vi "6509 Sensor Inputs.vi"(2 "error in":errorcluster, 3 "Enum":T1(ring)) -> (0 "error out":errorcluster, 1 "State":bool)   [LabVIEW 2014]
panel:
  out "task out":refnum<k21>
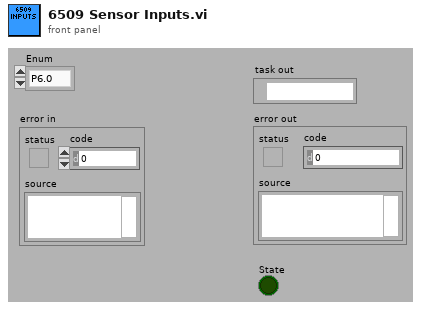
[diagram p1: front panel]
types:
  T1 = enum16{"P6.0", "P6.1", "P6.2", "P6.3", "P6.4", "P6.5", "P6.6", "P6.7", "P7.0", "P7.1", "P7.2", "P7.3", "P7.4", "P7.5", "P7.6", "P7.7", "P8.0", "P8.1", "P8.2", "P8.3", "P8.4", "P8.5", "P8.6", "P8.7", "P9.0", "P9.1", "P9.2", "P9.3", "P9.4", "P9.5", "P9.6", "P9.7", "11.0", "11.1", "11.2", "11.3", "11.4", "11.5", "11.6", "11.7", "Init"}
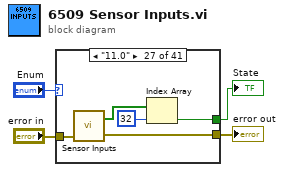
[diagram p0: block diagram]
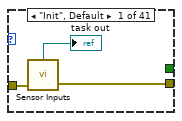
[diagram p2: hidden frame]
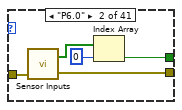
[diagram p3: hidden frame]
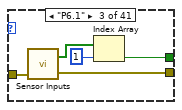
[diagram p4: hidden frame]
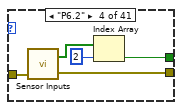
[diagram p5: hidden frame]
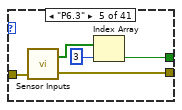
[diagram p6: hidden frame]
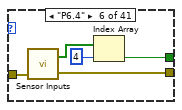
[diagram p7: hidden frame]
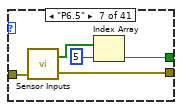
[diagram p8: hidden frame]
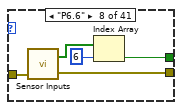
[diagram p9: hidden frame]
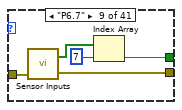
[diagram p10: hidden frame]
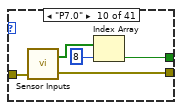
[diagram p11: hidden frame]
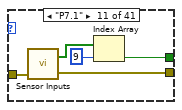
[diagram p12: hidden frame]
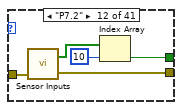
[diagram p13: hidden frame]
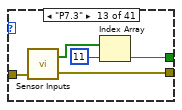
[diagram p14: hidden frame]
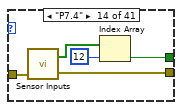
[diagram p15: hidden frame]
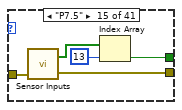
[diagram p16: hidden frame]
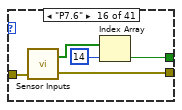
[diagram p17: hidden frame]
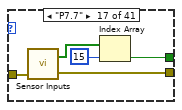
[diagram p18: hidden frame]
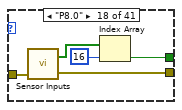
[diagram p19: hidden frame]
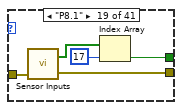
[diagram p20: hidden frame]
diagram:
  n1 = case shown="\"11.0\"" "Enum" {
    tunnel: "error in" -> [w7 w11 w15 w20 w23 w30 w35 w40 w45 w50 w55 w59 w65 w68 w75 w80 w85 w88 w95 w98 w103 w110 w113 w118 w123 w129 w134 w139 w144 w149 w154 w159 w164 w169 w175 w180 w184 w188 w194 w198 w204]
    tunnel: [w6 w10 w14 w19 w25 w28 w34 w39 w44 w49 w54 w60 w64 w70 w74 w79 w84 w90 w94 w100 w105 w109 w115 w120 w125 w130 w135 w140 w145 w150 w155 w160 w165 w170 w174 w179 w185 w190 w195 w200 w205] -> w2
    tunnel: [_ w8 w13 w18 w24 w29 w33 w38 w43 w48 w53 w58 w63 w69 w73 w78 w83 w89 w93 w99 w104 w108 w114 w119 w124 w128 w133 w138 w143 w148 w153 w158 w163 w168 w173 w178 w183 w189 w193 w199 w203] -> w1
    frame "Init", Default {
      n2 = call "Sensor Inputs.vi"("error in"=w7) -> ("error out"=w6:errorcluster, "task out"=→"task out":refnum<k21>)  [unwired: 2 in, 1 out]
    }
    frame "P6.0" {
      n3 = call "Sensor Inputs.vi"("error in"=w11) -> ("error out"=w10:errorcluster, "data"=w9:bool[])  [unwired: 2 in, 1 out]
      n4 = Index Array(array=w9, index=0) -> (element=w8:bool)
    }
    frame "P6.1" {
      n5 = call "Sensor Inputs.vi"("error in"=w15) -> ("error out"=w14:errorcluster, "data"=w16:bool[])  [unwired: 2 in, 1 out]
      n6 = Index Array(array=w16, index=1) -> (element=w13:bool)
    }
    frame "P6.2" {
      n7 = call "Sensor Inputs.vi"("error in"=w20) -> ("error out"=w19:errorcluster, "data"=w21:bool[])  [unwired: 2 in, 1 out]
      n8 = Index Array(array=w21, index=2) -> (element=w18:bool)
    }
    frame "P6.3" {
      n9 = call "Sensor Inputs.vi"("error in"=w23) -> ("error out"=w25:errorcluster, "data"=w26:bool[])  [unwired: 2 in, 1 out]
      n10 = Index Array(array=w26, index=3) -> (element=w24:bool)
    }
    frame "P6.4" {
      n11 = call "Sensor Inputs.vi"("error in"=w30) -> ("error out"=w28:errorcluster, "data"=w31:bool[])  [unwired: 2 in, 1 out]
      n12 = Index Array(array=w31, index=4) -> (element=w29:bool)
    }
    frame "P6.5" {
      n13 = call "Sensor Inputs.vi"("error in"=w35) -> ("error out"=w34:errorcluster, "data"=w36:bool[])  [unwired: 2 in, 1 out]
      n14 = Index Array(array=w36, index=5) -> (element=w33:bool)
    }
    frame "P6.6" {
      n15 = call "Sensor Inputs.vi"("error in"=w40) -> ("error out"=w39:errorcluster, "data"=w41:bool[])  [unwired: 2 in, 1 out]
      n16 = Index Array(array=w41, index=6) -> (element=w38:bool)
    }
    frame "P6.7" {
      n17 = call "Sensor Inputs.vi"("error in"=w45) -> ("error out"=w44:errorcluster, "data"=w46:bool[])  [unwired: 2 in, 1 out]
      n18 = Index Array(array=w46, index=7) -> (element=w43:bool)
    }
    frame "P7.0" {
      n19 = call "Sensor Inputs.vi"("error in"=w50) -> ("error out"=w49:errorcluster, "data"=w51:bool[])  [unwired: 2 in, 1 out]
      n20 = Index Array(array=w51, index=8) -> (element=w48:bool)
    }
    frame "P7.1" {
      n21 = call "Sensor Inputs.vi"("error in"=w55) -> ("error out"=w54:errorcluster, "data"=w56:bool[])  [unwired: 2 in, 1 out]
      n22 = Index Array(array=w56, index=9) -> (element=w53:bool)
    }
    frame "P7.2" {
      n23 = call "Sensor Inputs.vi"("error in"=w59) -> ("error out"=w60:errorcluster, "data"=w61:bool[])  [unwired: 2 in, 1 out]
      n24 = Index Array(array=w61, index=10) -> (element=w58:bool)
    }
    frame "P7.3" {
      n25 = call "Sensor Inputs.vi"("error in"=w65) -> ("error out"=w64:errorcluster, "data"=w66:bool[])  [unwired: 2 in, 1 out]
      n26 = Index Array(array=w66, index=11) -> (element=w63:bool)
    }
    frame "P7.4" {
      n27 = call "Sensor Inputs.vi"("error in"=w68) -> ("error out"=w70:errorcluster, "data"=w71:bool[])  [unwired: 2 in, 1 out]
      n28 = Index Array(array=w71, index=12) -> (element=w69:bool)
    }
    frame "P7.5" {
      n29 = call "Sensor Inputs.vi"("error in"=w75) -> ("error out"=w74:errorcluster, "data"=w76:bool[])  [unwired: 2 in, 1 out]
      n30 = Index Array(array=w76, index=13) -> (element=w73:bool)
    }
    frame "P7.6" {
      n31 = call "Sensor Inputs.vi"("error in"=w80) -> ("error out"=w79:errorcluster, "data"=w81:bool[])  [unwired: 2 in, 1 out]
      n32 = Index Array(array=w81, index=14) -> (element=w78:bool)
    }
    frame "P7.7" {
      n33 = call "Sensor Inputs.vi"("error in"=w85) -> ("error out"=w84:errorcluster, "data"=w86:bool[])  [unwired: 2 in, 1 out]
      n34 = Index Array(array=w86, index=15) -> (element=w83:bool)
    }
    frame "P8.0" {
      n35 = call "Sensor Inputs.vi"("error in"=w88) -> ("error out"=w90:errorcluster, "data"=w91:bool[])  [unwired: 2 in, 1 out]
      n36 = Index Array(array=w91, index=16) -> (element=w89:bool)
    }
    frame "P8.1" {
      n37 = call "Sensor Inputs.vi"("error in"=w95) -> ("error out"=w94:errorcluster, "data"=w96:bool[])  [unwired: 2 in, 1 out]
      n38 = Index Array(array=w96, index=17) -> (element=w93:bool)
    }
    frame "P8.2" {
      n39 = call "Sensor Inputs.vi"("error in"=w98) -> ("error out"=w100:errorcluster, "data"=w101:bool[])  [unwired: 2 in, 1 out]
      n40 = Index Array(array=w101, index=18) -> (element=w99:bool)
    }
    frame "P8.3" {
      n41 = call "Sensor Inputs.vi"("error in"=w103) -> ("error out"=w105:errorcluster, "data"=w106:bool[])  [unwired: 2 in, 1 out]
      n42 = Index Array(array=w106, index=19) -> (element=w104:bool)
    }
    frame "P8.4" {
      n43 = call "Sensor Inputs.vi"("error in"=w110) -> ("error out"=w109:errorcluster, "data"=w111:bool[])  [unwired: 2 in, 1 out]
      n44 = Index Array(array=w111, index=20) -> (element=w108:bool)
    }
    frame "P8.5" {
      n45 = call "Sensor Inputs.vi"("error in"=w113) -> ("error out"=w115:errorcluster, "data"=w116:bool[])  [unwired: 2 in, 1 out]
      n46 = Index Array(array=w116, index=21) -> (element=w114:bool)
    }
    frame "P8.6" {
      n47 = call "Sensor Inputs.vi"("error in"=w118) -> ("error out"=w120:errorcluster, "data"=w121:bool[])  [unwired: 2 in, 1 out]
      n48 = Index Array(array=w121, index=22) -> (element=w119:bool)
    }
    frame "P8.7" {
      n49 = call "Sensor Inputs.vi"("error in"=w123) -> ("error out"=w125:errorcluster, "data"=w126:bool[])  [unwired: 2 in, 1 out]
      n50 = Index Array(array=w126, index=23) -> (element=w124:bool)
    }
    frame "P9.0" {
      n51 = call "Sensor Inputs.vi"("error in"=w129) -> ("error out"=w130:errorcluster, "data"=w131:bool[])  [unwired: 2 in, 1 out]
      n52 = Index Array(array=w131, index=24) -> (element=w128:bool)
    }
    frame "11.0" {
      n53 = call "Sensor Inputs.vi"("error in"=w134) -> ("error out"=w135:errorcluster, "data"=w136:bool[])  [unwired: 2 in, 1 out]
      n54 = Index Array(array=w136, index=32) -> (element=w133:bool)
    }
    frame "11.1" {
      n55 = call "Sensor Inputs.vi"("error in"=w139) -> ("error out"=w140:errorcluster, "data"=w141:bool[])  [unwired: 2 in, 1 out]
      n56 = Index Array(array=w141, index=33) -> (element=w138:bool)
    }
    frame "11.2" {
      n57 = call "Sensor Inputs.vi"("error in"=w144) -> ("error out"=w145:errorcluster, "data"=w146:bool[])  [unwired: 2 in, 1 out]
      n58 = Index Array(array=w146, index=34) -> (element=w143:bool)
    }
    frame "11.3" {
      n59 = call "Sensor Inputs.vi"("error in"=w149) -> ("error out"=w150:errorcluster, "data"=w151:bool[])  [unwired: 2 in, 1 out]
      n60 = Index Array(array=w151, index=35) -> (element=w148:bool)
    }
    frame "11.4" {
      n61 = call "Sensor Inputs.vi"("error in"=w154) -> ("error out"=w155:errorcluster, "data"=w156:bool[])  [unwired: 2 in, 1 out]
      n62 = Index Array(array=w156, index=36) -> (element=w153:bool)
    }
    frame "11.5" {
      n63 = call "Sensor Inputs.vi"("error in"=w159) -> ("error out"=w160:errorcluster, "data"=w161:bool[])  [unwired: 2 in, 1 out]
      n64 = Index Array(array=w161, index=37) -> (element=w158:bool)
    }
    frame "11.6" {
      n65 = call "Sensor Inputs.vi"("error in"=w164) -> ("error out"=w165:errorcluster, "data"=w166:bool[])  [unwired: 2 in, 1 out]
      n66 = Index Array(array=w166, index=38) -> (element=w163:bool)
    }
    frame "11.7" {
      n67 = call "Sensor Inputs.vi"("error in"=w169) -> ("error out"=w170:errorcluster, "data"=w171:bool[])  [unwired: 2 in, 1 out]
      n68 = Index Array(array=w171, index=39) -> (element=w168:bool)
    }
    frame "P9.1" {
      n69 = call "Sensor Inputs.vi"("error in"=w175) -> ("error out"=w174:errorcluster, "data"=w176:bool[])  [unwired: 2 in, 1 out]
      n70 = Index Array(array=w176, index=25) -> (element=w173:bool)
    }
    frame "P9.2" {
      n71 = call "Sensor Inputs.vi"("error in"=w180) -> ("error out"=w179:errorcluster, "data"=w181:bool[])  [unwired: 2 in, 1 out]
      n72 = Index Array(array=w181, index=27) -> (element=w178:bool)
    }
    frame "P9.3" {
      n73 = call "Sensor Inputs.vi"("error in"=w184) -> ("error out"=w185:errorcluster, "data"=w186:bool[])  [unwired: 2 in, 1 out]
      n74 = Index Array(array=w186, index=28) -> (element=w183:bool)
    }
    frame "P9.4" {
      n75 = call "Sensor Inputs.vi"("error in"=w188) -> ("error out"=w190:errorcluster, "data"=w191:bool[])  [unwired: 2 in, 1 out]
      n76 = Index Array(array=w191, index=29) -> (element=w189:bool)
    }
    frame "P9.5" {
      n77 = call "Sensor Inputs.vi"("error in"=w194) -> ("error out"=w195:errorcluster, "data"=w196:bool[])  [unwired: 2 in, 1 out]
      n78 = Index Array(array=w196, index=30) -> (element=w193:bool)
    }
    frame "P9.6" {
      n79 = call "Sensor Inputs.vi"("error in"=w198) -> ("error out"=w200:errorcluster, "data"=w201:bool[])  [unwired: 2 in, 1 out]
      n80 = Index Array(array=w201, index=31) -> (element=w199:bool)
    }
    frame "P9.7" {
      n81 = call "Sensor Inputs.vi"("error in"=w204) -> ("error out"=w205:errorcluster, "data"=w206:bool[])  [unwired: 2 in, 1 out]
      n82 = Index Array(array=w206, index=31) -> (element=w203:bool)
    }
  }
  "error out" <- w2
  "State" <- w1
